vi "Save_to_Project.vi"(8 "error in (no error)":errorcluster, 9 "index in":string, 10 "buildObject":T2, 11 "IB_Shortcut in":refnum<class "IB_Shortcut.lvclass">) -> (0 "error out":errorcluster, 1 "index out":string, 2 "buildObject out":T2, 3 "IB_Shortcut out":refnum<class "IB_Shortcut.lvclass">)   [LabVIEW 2020, in "IB_Shortcut.lvclass"]
uses:
  <vilib>/AppBuilder/IB_Classes/Shortcut/IB_Shortcut.lvclass
  <vilib>/AppBuilder/IB_Classes/Shortcut/IB_Shortcut.lvclass/IB_Shortcut.ctl
  <vilib>/AppBuilder/IB_RW_Project/IB_RW_Project_PropBag_Action.ctl
  <resource>/Framework/Providers/API/ItemRef.ctl
  <vilib>/AppBuilder/IB_RW_Project/IB_RW_Project_Shortcut_Data.ctl
panel:
  in  "data":T1
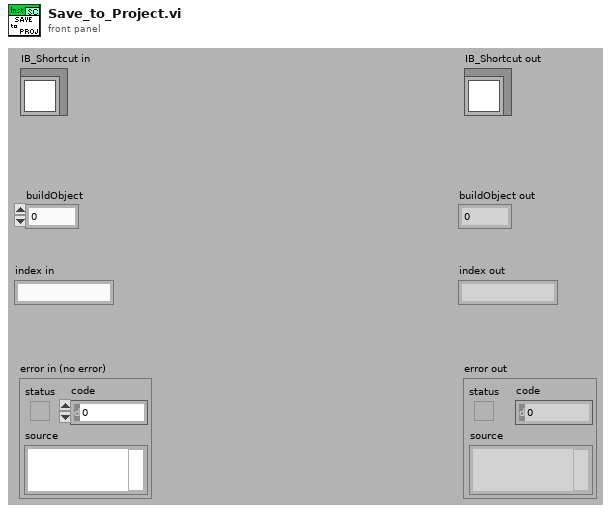
[diagram p1: front panel]
types:
  T1 = typedef "IB_RW_Project_Shortcut_Data.ctl" = cluster{"name":string, "destIndex":i32, "subDir":string}
  T2 = typedef "ItemRef.ctl" = u64
  T3 = typedef "IB_RW_Project_PropBag_Action.ctl" = enum16{"read", "write", "clear", "readPrevious", "writePrevious", "clearPrevious"}
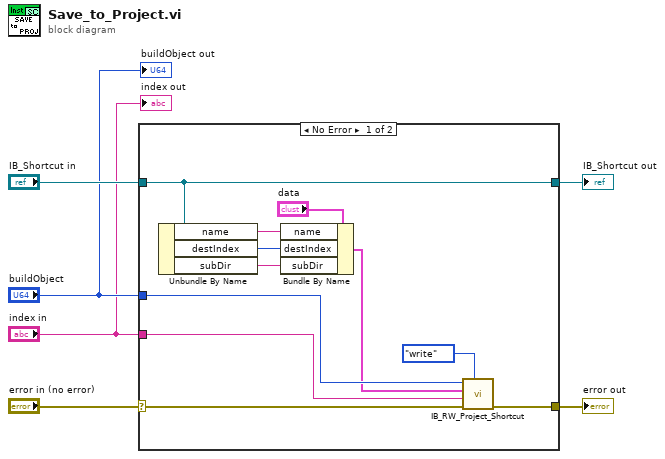
[diagram p0: block diagram]
diagram:
  n1 = case shown="No Error" "error in (no error)" {
    selector: "error in (no error)" -> [w12 w19]
    tunnel: [w11 w19] -> w5
    tunnel: [w17 w18] -> w3
    tunnel: "IB_Shortcut in" -> [w17 w18]
    tunnel: "buildObject" -> [w10 _]
    tunnel: "index in" -> [w13 _]
    frame No Error {
      n2 = Unbundle By Name(w17) -> ("name"=w15:string, "destIndex"=w7:i32, "subDir"=w14:string)
      n3 = Bundle By Name(cluster="data", "name"=w15, "destIndex"=w7, "subDir"=w14) -> (w9:T1)
      n4 = call <vilib>:"IB_RW_Project_Shortcut.vi"("action"=IB_RW_Project_PropBag_Action."write", "error in (no error)"=w12, "index in"=w13, "dataSource in"=w9, "buildObject"=w10) -> ("error out"=w11:errorcluster)  [unwired: 6 out]
    }
    frame Error {
    }
  }
  "error out" <- w5
  "IB_Shortcut out" <- w3
  "buildObject out" <- "buildObject"
  "index out" <- "index in"
